vi "UtilityDIO.vi"(1 "Immediate":bool, 2 "Digital Output":u16 format="%.0x") -> (0 "Digital Input":u16 format="%.0x")   [LabVIEW 2014]
panel:
  in  "Read":bool caption="Exit"
  in  "Write":bool caption="Exit"
  in  "Exit":bool
  in  "Digital Value":bool[](array[boolean])
  # "D0"
  # "D1"
  # "D2"
  # "D3"
  # "D4"
  # "D5"
  # "D6"
  # "D7"
  # "D8"
  # "D9"
  # "D10"
  # "D11"
  # "D12"
  # "D13"
  # "D14"
  # "D15"
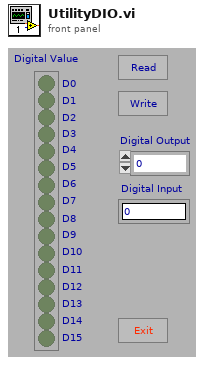
[diagram p1: front panel]
types:
  T1 = enum32{"not used", "PCI_BOARD", "TIMING_BOARD", "UTILITY_BOARD"}
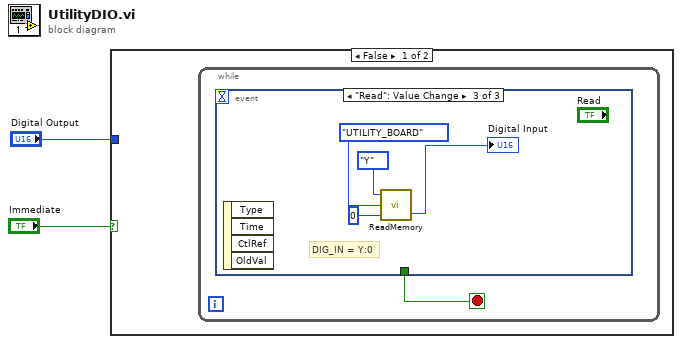
[diagram p0: block diagram]
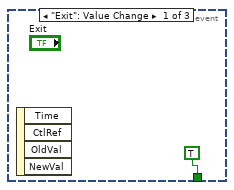
[diagram p2: hidden frame]
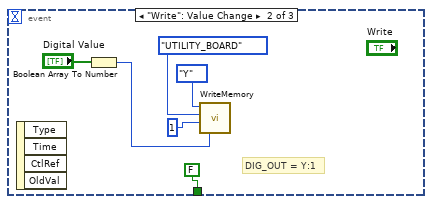
[diagram p3: hidden frame]
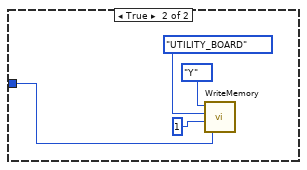
[diagram p4: hidden frame]
diagram:
  n1 = case shown="False" "Immediate" {
    tunnel: "Digital Output" -> [_ w15]
    frame False {
      n2 = while {
        stop <- w3 stop-if-true
        n3 = event shown="[2] \"Read\": Value Change" {
          selector: _ -> [_ _ _]
          dyn-events: _ -> [_ _ _]
          timeout: _ -> [_ _ _]
          tunnel: [TRUE FALSE _] -> w3
          event "Exit": Value Change {
            n4 = event-data() -> ()  [unwired: 1 in, 4 out]
          }
          event "Write": Value Change {
            # "DIG_OUT = Y:1"
            n5 = event-data() -> ()  [unwired: 1 in, 4 out]
            n6 = Boolean Array To Number(Boolean array="Digital Value") -> (number=w5:u32)
            n7 = call "WriteMemory.vi"("Value"=w5, "Address"=1 ("address"), "Board"=T1."UTILITY_BOARD" ("board"), "Type"=enum16{"X", "Y", "P", "R", "D"}."Y") -> ()  [unwired: 1 out]
          }
          event "Read": Value Change {
            # "DIG_IN = Y:0"
            n8 = event-data() -> ()  [unwired: 1 in, 4 out]
            n9 = call "ReadMemory.vi"("Address"=0 ("address"), "Board"=T1."UTILITY_BOARD" ("board"), "Type"=enum16{"X", "Y", "P", "R", "D"}."Y") -> ("Value"=→"Digital Input":i32)  [unwired: 1 out]
          }
        }
      }
    }
    frame True {
      n10 = call "WriteMemory.vi"("Value"=w15, "Address"=1 ("address"), "Board"=T1."UTILITY_BOARD" ("board"), "Type"=enum16{"X", "Y", "P", "R", "D"}."Y") -> ()  [unwired: 1 out]
    }
  }
